vi "Start Driving with Limelight.vi"(11 "Drive with Limelight":bool) -> ()   [LabVIEW 2020]
uses:
  Robot Global Data.vi
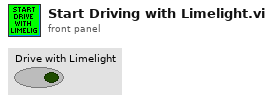
[diagram p1: front panel]
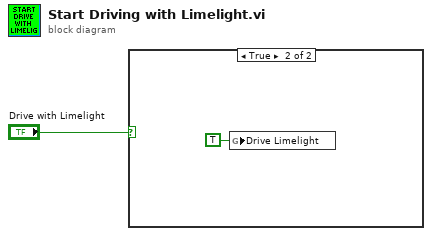
[diagram p0: block diagram]
diagram:
  n1 = case shown="True" "Drive with Limelight" {
    frame False {
    }
    frame True {
      n2 = global write "Robot Global Data.vi" "Drive Limelight"(TRUE ("Drive Limelight")) -> ()
    }
  }
